vi "Add Table.vi"(5 "Adr":string, 7 "Index":i32, 8 "error in":errorcluster, 9 "Data_Str":string[][](array[string]), 10 "Headers":string[](array[string]), 11 "XLS in":refnum<class "XLS.lvclass">) -> (0 "error out":errorcluster, 3 "XLS out":refnum<class "XLS.lvclass">)   [LabVIEW 2017, in "Report_lib.lvlib" / "XLS.lvclass"]
doc: "This method Add to xls report a table - \n2D string array with separated Headers.\nCoords pre-defined and post-defined after\nadd a table"
uses:
  XLS.lvclass
  XLS.lvclass/XLS.ctl
  <vilib>/Utility/NIReport.llb/Append Text Table to Report (wrap).vi
  <vilib>/Utility/NIReport.llb/NI_report.lvclass
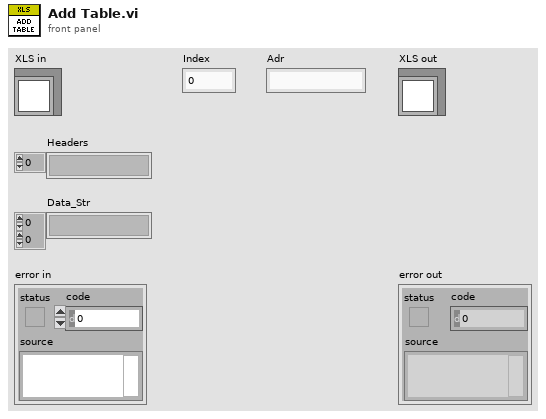
[diagram p1: front panel]
types:
  T1 = cluster{"position":cluster{"row":i32, "column":i32}, "Adr":string, "Index":string}
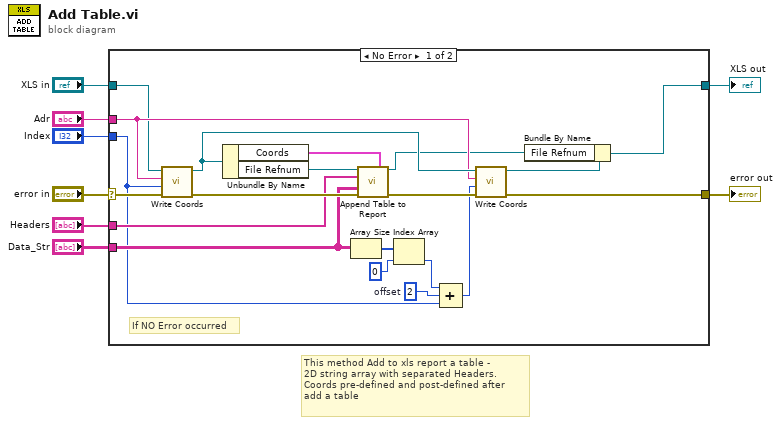
[diagram p0: block diagram]
diagram:
  # "This method Add to xls report a table - \n2D string array with separated Headers.\nCoords pre-defined and post-defined after\nadd a table"
  n1 = case shown="No Error" "error in" {
    selector: "error in" -> [w24 w30]
    tunnel: [w18 w30] -> w7
    tunnel: [w9 w29] -> w5
    tunnel: "XLS in" -> [w10 w29]
    tunnel: "Adr" -> [w13 _]
    tunnel: "Index" -> [w15 _]
    tunnel: "Headers" -> [w22 _]
    tunnel: "Data_Str" -> [w21 _]
    frame No Error {
      w17 = 2  # offset
      # "If NO Error occurred"
      n2 = call "Write Coords.vi"("error in"=w24, "Index"=w15, "Adr"=w13, "XLS in"=w10) -> ("error out"=w23:errorcluster, "XLS out"=w19:refnum<class "XLS.lvclass">)  [unwired: 6 in]
      n3 = Unbundle By Name(w19) -> ("Coords"=w25:T1, "File Refnum"=w26:refnum<class "NI_report.lvclass">)
      n4 = Array Size(array=w21) -> (size(s)=w28:i32[])
      n5 = call-poly <vilib>:"Append Table to Report.vi"("report in"=w26, "MS Office parameters"=w25, "column headers"=w22, "text data"=w21, "error in (no error)"=w23) -> ("report out"=w11:refnum<class "NI_report.lvclass">, "error out"=w20:errorcluster)  [unwired: 7 in, 2 out]
      n6 = Index Array(array=w28, index=0) -> (element=w16:i32)
      n7 = Compound Arithmetic op=ADD(w16, w17, w15) -> (w14:i32)
      n8 = call "Write Coords.vi"("error in"=w20, "Index"=w14, "Adr"=w13, "XLS in"=w19) -> ("error out"=w18:errorcluster, "XLS out"=w12:refnum<class "XLS.lvclass">)  [unwired: 6 in]
      n9 = Bundle By Name(cluster=w12, "File Refnum"=w11) -> (w9:refnum<class "XLS.lvclass">)
    }
    frame Error {
    }
  }
  "error out" <- w7
  "XLS out" <- w5
